vi "Steplogic.vi"(8 "StepSize":u32 format="%018b", 9 "act Step 18 Bit":u32=16 format="%018b", 11 "Stop":u32 format="%018b") -> (1 "Next Step":u32=16 format="%0d", 3 "Done":bool)   [LabVIEW 2014]
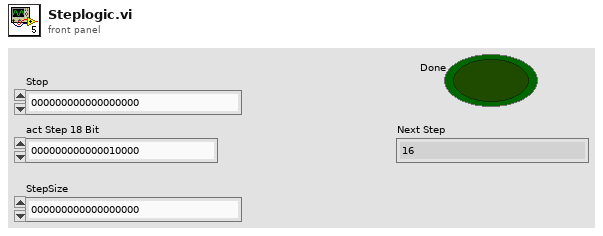
[diagram p1: front panel]
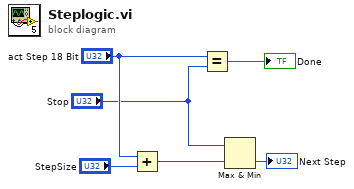
[diagram p0: block diagram]
diagram:
  n1 = Add(x="act Step 18 Bit", y="StepSize") -> (x+y=w3:u32)
  n2 = Equal?(x="act Step 18 Bit", y="Stop") -> (x = y?=→"Done":bool)
  n3 = Max & Min(x="Stop", y=w3) -> (min(x,y)=→"Next Step":u32)  [unwired: 1 out]
